vi "runtest check for empty steps.vi"(9 "No Steps? (f)":bool, 11 "error in (no error)":errorcluster) -> (3 "error out":errorcluster)   [LabVIEW 2011]
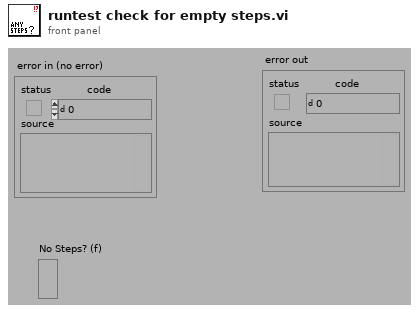
[diagram p1: front panel]
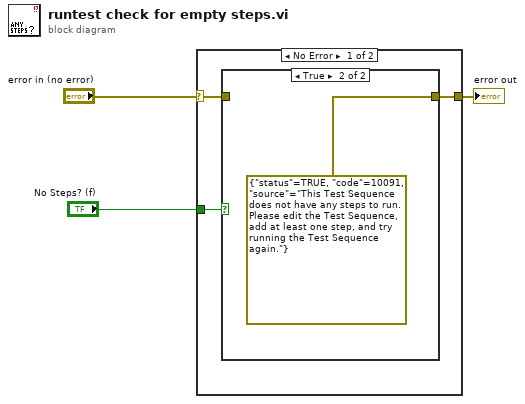
[diagram p0: block diagram]
diagram:
  n1 = case shown="No Error" "error in (no error)" {
    selector: "error in (no error)" -> [w4 w9]
    tunnel: [w6 w9] -> w2
    tunnel: "No Steps? (f)" -> [w5 _]
    frame No Error {
      n2 = case shown="True" w5 {
        tunnel: [w7 errorcluster {"status"=TRUE, "code"=10091, "source"="This Test Sequence does not have any steps to run.  Please edit the Test Sequence, add at least one step, and try running the Test Sequence again."} ("error out")] -> w6
        tunnel: w4 -> [w7 _]
        frame False {
        }
        frame True {
        }
      }
    }
    frame Error {
    }
  }
  "error out" <- w2
